vi "TDMS Merge Utility.vi"() -> ()   [LabVIEW 2011]
uses:
  <userlib>/_OpenG.lib/file/file.llb/Strip Path - Traditional__ogtk.vi
  <userlib>/_OpenG.lib/file/file.llb/Build Path - Traditional__ogtk.vi
  <userlib>/_OpenG.lib/file/file.llb/File Exists - Scalar__ogtk.vi
  <userlib>/_OpenG.lib/file/file.llb/Convert File Extension (Path)__ogtk.vi
panel:
  out "of":i32
  out "Files Processed":i32
  out "Progress Bar":u8(slide)=100 scale=0.0..100.0
  out "error out":errorcluster
  in  "Data Directory":path=path "\\\\10.196.0.53\\e$/Spartan/data/TDM"
  in  "Directory to Move":path=path "\\\\10.196.0.53\\e$/Spartan/data/xtdm"
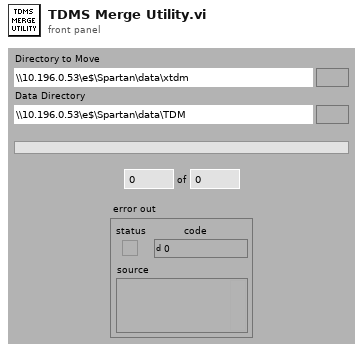
[diagram p1: front panel]
types:
  T1 = enum16{"open", "open or create", "create or replace", "create", "open (read-only)"}
  T2 = cluster{dbl, "tdms file out":refnum<k34>, string}
  T3 = cluster{dbl, "tdms file out":refnum<k34>, string}[]
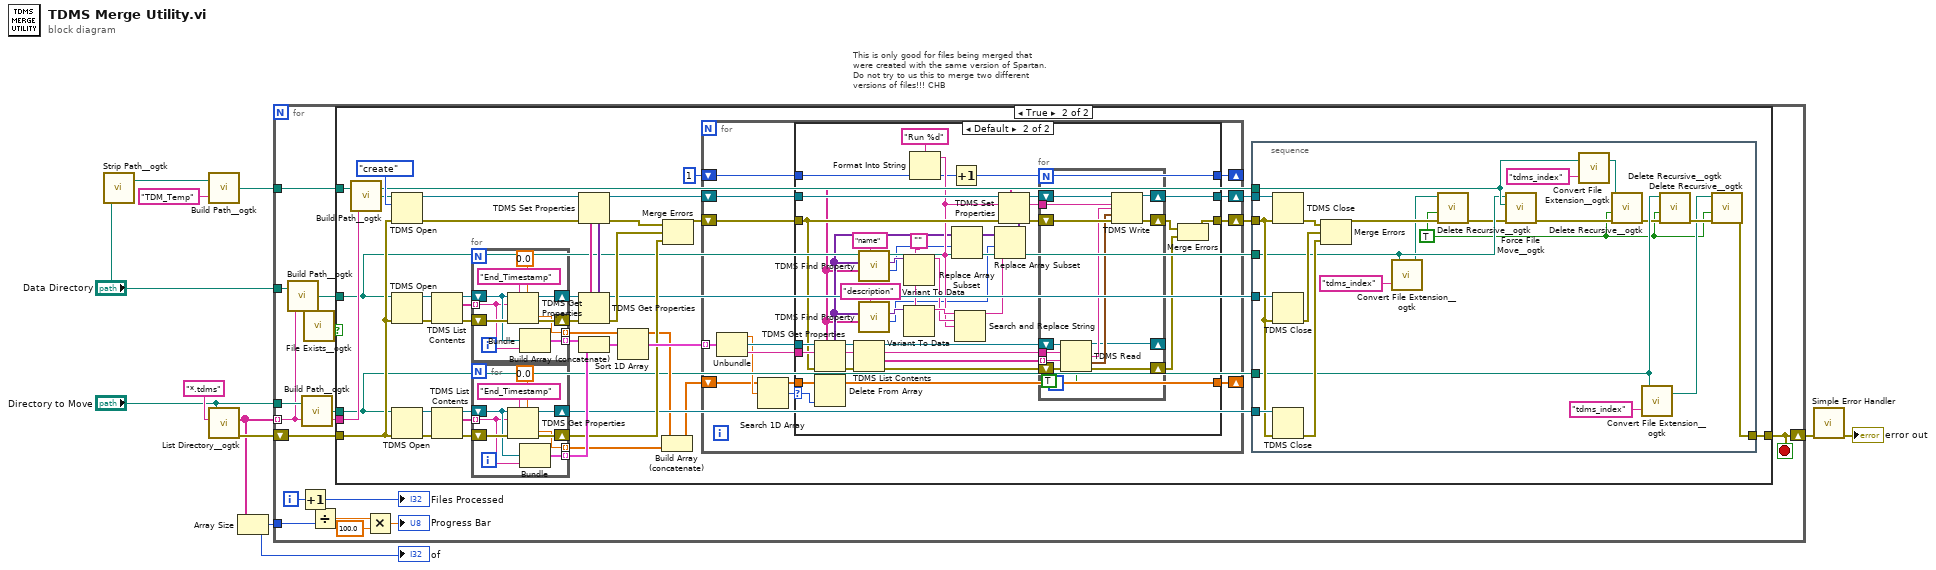
[diagram p0: block diagram]
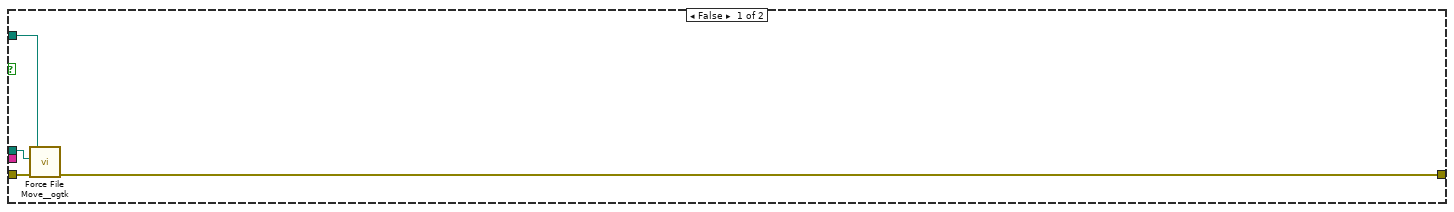
[diagram p2: hidden frame]
diagram:
  # "This is only good for files being merged that\nwere created with the same version of Spartan.\nDo not try to us this to merge two different\nversions of files!!! CHB"
  n1 = call-poly <userlib>:"Strip Path__ogtk.vi"("path"="Data Directory") -> ("stripped path"=w3:path)  [unwired: 1 out]
  n2 = call-poly <userlib>:"Build Path__ogtk.vi"("name or relative path"="TDM_Temp" ("Relative Path (\"\" - Folder)"), "base path"=w3) -> ("appended path"=w7:path)
  n3 = call <userlib>:"List Directory__ogtk.vi"("pattern"="*.tdms", "directory path"="Directory to Move") -> ("error out"=w10:errorcluster, "file names"=w2:string[])  [unwired: 2 in, 2 out]
  n4 = Array Size(array=w2) -> (size(s)=w1:i32)
  "of" <- w1
  n5 = for {
    shift-right: [w21] -> w6
    shift-left: w10 -> [w26]
    tunnel: w2 -> [w13] mode=indexing
    tunnel: "Data Directory" -> [w25]
    tunnel: "Directory to Move" -> [w14]
    tunnel: w7 -> [w22]
    tunnel: w1 -> [w18]
    i -> [w20]
    stop <- w21 stop-if-true
    n6 = call-poly <userlib>:"Build Path__ogtk.vi"("name or relative path"=w13, "base path"=w25) -> ("appended path"=w24:path)
    n7 = Increment(x=w20) -> (x+1=w19:i32)
    "Files Processed" <- w19
    n8 = call-poly <userlib>:"Build Path__ogtk.vi"("name or relative path"=w13, "base path"=w14) -> ("appended path"=w12:path)
    n9 = call-poly <userlib>:"File Exists__ogtk.vi"("file path"=w24) -> ("exists"=w23:bool)  [unwired: 6 in, 1 out]
    n10 = Divide(x=w19, y=w18) -> (x/y=w17:dbl)
    n11 = case shown="True" w23 {
      tunnel: w26 -> [w30 w66]
      tunnel: w13 -> [_ w64]
      tunnel: w24 -> [w29 w38]
      tunnel: [w28 w37] -> w21
      tunnel: w22 -> [_ w39]
      tunnel: w12 -> [w27 w31]
      frame False {
        n12 = call <userlib>:"Force File Move__ogtk.vi"("error in (no error)"=w30, "source"=w27, "target"=w29) -> ("error out"=w28:errorcluster)  [unwired: 3 in, 1 out]
      }
      frame True {
        n13 = call-poly <userlib>:"Build Path__ogtk.vi"("name or relative path"=w64, "base path"=w39) -> ("appended path"=w36:path)
        n14 = TDMS Open(8:w66, 10:T1."create" ("operation (0:open)"), 11:w36) -> (0:w53:errorcluster, 3:w52:refnum<k34>)  [unwired: 3 in]
        n15 = TDMS Open(8:w66, 11:w38) -> (0:w63:errorcluster, 3:w62:refnum<k34>)  [unwired: 4 in]
        n16 = TDMS Open(8:w66, 11:w31) -> (0:w71:errorcluster, 3:w70:refnum<k34>)  [unwired: 4 in]
        n17 = TDMS List Contents(4:w63, 7:w62) -> (0:w61:errorcluster, 2:w59:string[], 3:w60:refnum<k34>)  [unwired: 1 in, 1 out]
        n18 = TDMS List Contents(4:w71, 7:w70) -> (0:w69:errorcluster, 2:w67:string[], 3:w68:refnum<k34>)  [unwired: 1 in, 1 out]
        n19 = for {
          shift-right: [w171] -> w54
          shift-left: w61 -> [w173]
          shift-right: [w170] -> w55
          shift-left: w60 -> [w169]
          tunnel: w59 -> [w168] mode=indexing
          tunnel: [w167] -> w58 mode=indexing
          tunnel: [w165] -> w35 mode=indexing
          n20 = TDMS Get Properties(5:0.0, 7:"End_Timestamp" ("pattern"), 8:w173, 10:w168, 11:w169) -> (0:w171:errorcluster, 3:w170:refnum<k34>, 4:w165:dbl)  [unwired: 1 in, 3 out]
          n21 = Bundle(w165, "tdms file out"=w169, w168) -> (w167:T2)  [unwired: 1 in]
        }
        n22 = for {
          shift-right: [w180] -> w46
          shift-left: w69 -> [w182]
          shift-right: [w179] -> w40
          shift-left: w68 -> [w178]
          tunnel: w67 -> [w177] mode=indexing
          tunnel: [w176] -> w57 mode=indexing
          tunnel: [w174] -> w34 mode=indexing
          n23 = TDMS Get Properties(5:0.0, 7:"End_Timestamp" ("pattern"), 8:w182, 10:w177, 11:w178) -> (0:w180:errorcluster, 3:w179:refnum<k34>, 4:w174:dbl)  [unwired: 1 in, 3 out]
          n24 = Bundle(w174, "tdms file out"=w178, w177) -> (w176:T2)  [unwired: 1 in]
        }
        n25 = TDMS Get Properties(8:w54, 11:w55) -> (0:w47:errorcluster, 3:w41:refnum<k34>, 4:w50:variant[], 6:w51:string[])  [unwired: 4 in, 2 out]
        n26 = TDMS Set Properties(5:w50, 7:w51, 8:w53, 11:w52) -> (0:w45:errorcluster, 3:w48:refnum<k34>)  [unwired: 2 in, 2 out]
        n27 = Build Array (concatenate)(w58, w57) -> (w56:T3)
        n28 = Sort 1D Array(array=w56) -> (sorted array=w49:T3)
        n29 = Build Array (concatenate)(w35, w34) -> (w33:dbl[])
        n30 = Merge Errors(w45, w47, w46) -> (w44:errorcluster)
        n31 = for {
          tunnel: w49 -> [w107] mode=indexing
          shift-right: [w102] -> w42
          shift-left: w44 -> [w104]
          shift-right: [w101] -> w43
          shift-left: w48 -> [w103]
          shift-right: [w98] -> _
          shift-left: w33 -> [w97]
          shift-right: [w95] -> _
          shift-left: 1 -> [w96]
          n32 = Unbundle(w107) -> (w100:dbl, "tdms file out"=w106:refnum<k34>, w105:string)
          n33 = Search 1D Array(1D array=w97, element=w100) -> (index of element=w99:i32)  [unwired: 1 in]
          n34 = case shown="Default" w99 {
            selector: w99 -> [_ w114]
            tunnel: w106 -> [_ w149]
            tunnel: w105 -> [_ w148]
            tunnel: w104 -> [w111 w147]
            tunnel: w103 -> [w110 w146]
            tunnel: [w111 w134] -> w102
            tunnel: [w110 w132] -> w101
            tunnel: [w109 w115] -> w98
            tunnel: w97 -> [w109 w116]
            tunnel: w96 -> [w108 w113]
            tunnel: [w108 w112] -> w95
            frame -1 {
            }
            frame Default {
              w126 = ""
              n35 = TDMS Get Properties(8:w147, 10:w148, 11:w149) -> (0:w145:errorcluster, 2:w143:string, 3:w144:refnum<k34>, 4:w123:variant[], 6:w122:string[])  [unwired: 3 in, 1 out]
              n36 = Delete From Array(array=w116, index=w114) -> (array with subset deleted=w115:dbl[])  [unwired: 1 in, 1 out]
              n37 = TDMS List Contents(4:w145, 6:w143, 7:w144) -> (0:w141:errorcluster, 1:w139:string[], 2:w140:string, 3:w142:refnum<k34>)
              n38 = call "TDMS Find Property.vi"("Property Name"="name", "Property Names"=w122, "Property Values"=w123) -> ("Index"=w120:i32, "Property Value"=w127:variant)  [unwired: 4 out]
              n39 = call "TDMS Find Property.vi"("Property Name"="description", "Property Names"=w122, "Property Values"=w123) -> ("Index"=w119:i32, "Property Value"=w129:variant)  [unwired: 4 out]
              n40 = Variant To Data(type=w126, Variant=w127) -> (data=w125:string)  [unwired: 1 in, 1 out]
              n41 = Variant To Data(type=w126, Variant=w129) -> (data=w128:string)  [unwired: 1 in, 1 out]
              n42 = Format Into String(format string="Run %d", w113) -> (resulting string=w124:string)  [unwired: 2 in, 1 out]
              n43 = Increment(x=w113) -> (x+1=w112:i32)
              n44 = Replace Array Subset(array=w123, new element=w124, index=w120) -> (w121:variant[])
              n45 = Search and Replace String(input string=w128, search string=w125, replace string=w124) -> (result string=w118:string)  [unwired: 5 in, 3 out]
              n46 = Replace Array Subset(array=w121, new element=w118, index=w119) -> (w117:variant[])
              n47 = TDMS Set Properties(5:w117, 7:w122, 8:w147, 10:w124, 11:w146) -> (0:w138:errorcluster, 2:w136:string, 3:w137:refnum<k34>)  [unwired: 1 in, 1 out]
              n48 = for {
                shift-right: [w155] -> _
                shift-left: w142 -> [w164]
                shift-right: [w154] -> w133
                shift-left: w141 -> [w163]
                tunnel: w140 -> [w162]
                tunnel: w139 -> [w161] mode=indexing
                shift-right: [w153] -> w132
                shift-left: w137 -> [w159]
                shift-right: [w152] -> w135
                shift-left: w138 -> [w160]
                tunnel: w136 -> [w158]
                n49 = TDMS Read(0:w164, 5:w162, 7:w161, 11:w163, 13:TRUE ("return channels in file order? (F)")) -> (4:w155:refnum<k34>, 8:w157:string, 10:w156:waveform(dbl), 15:w154:errorcluster)  [unwired: 3 in, 2 out]
                n50 = TDMS Write(0:w159, 5:w158, 7:w157, 9:w156, 11:w160) -> (4:w153:refnum<k34>, 15:w152:errorcluster)  [unwired: 1 in, 2 out]
              }
              n51 = Merge Errors(w135, w133) -> (w134:errorcluster)
            }
          }
        }
        n52 = stacked-sequence {
          tunnel: w43 -> [w92]
          tunnel: w42 -> [w91]
          tunnel: w41 -> [w94]
          tunnel: w40 -> [w93]
          tunnel: w36 -> [w82]
          tunnel: w38 -> [w76]
          tunnel: w31 -> [w87]
          tunnel: [w78] -> w37
          frame #0 {
            w72 = TRUE ("Ignore Read-Only? (FALSE)")
            n53 = TDMS Close(8:w91, 11:w92) -> (0:w90:errorcluster)  [unwired: 1 out]
            n54 = TDMS Close(8:w91, 11:w94) -> (0:w89:errorcluster)  [unwired: 1 out]
            n55 = TDMS Close(8:w91, 11:w93) -> (0:w88:errorcluster)  [unwired: 1 out]
            n56 = Merge Errors(w90, w89, w88) -> (w75:errorcluster)
            n57 = call-poly <userlib>:"Convert File Extension__ogtk.vi"("new ending (none)"="tdms_index", "file name"=w76) -> ("new filename"=w73:path)  [unwired: 1 out]
            n58 = call <userlib>:"Delete Recursive__ogtk.vi"("error in (no error)"=w75, "Ignore Read-Only? (FALSE)"=w72, "Path"=w73) -> ("error out"=w74:errorcluster)  [unwired: 7 in, 1 out]
            n59 = call <userlib>:"Force File Move__ogtk.vi"("error in (no error)"=w74, "source"=w82, "target"=w76) -> ("error out"=w85:errorcluster)  [unwired: 3 in, 1 out]
            n60 = call-poly <userlib>:"Convert File Extension__ogtk.vi"("new ending (none)"="tdms_index", "file name"=w82) -> ("new filename"=w81:path)  [unwired: 1 out]
            n61 = call <userlib>:"Delete Recursive__ogtk.vi"("error in (no error)"=w85, "Ignore Read-Only? (FALSE)"=w72, "Path"=w81) -> ("error out"=w84:errorcluster)  [unwired: 7 in, 1 out]
            n62 = call-poly <userlib>:"Convert File Extension__ogtk.vi"("new ending (none)"="tdms_index", "file name"=w87) -> ("new filename"=w79:path)  [unwired: 1 out]
            n63 = call <userlib>:"Delete Recursive__ogtk.vi"("error in (no error)"=w84, "Ignore Read-Only? (FALSE)"=w72, "Path"=w87) -> ("error out"=w80:errorcluster)  [unwired: 7 in, 1 out]
            n64 = call <userlib>:"Delete Recursive__ogtk.vi"("error in (no error)"=w80, "Ignore Read-Only? (FALSE)"=w72, "Path"=w79) -> ("error out"=w78:errorcluster)  [unwired: 7 in, 1 out]
          }
        }
      }
    }
    n65 = Multiply(x=w17, y=100.0) -> (x*y=→"Progress Bar":dbl)
  }
  n66 = call <vilib>:"Simple Error Handler.vi"("error in (no error)"=w6) -> ("error out"=→"error out":errorcluster)  [unwired: 4 in, 4 out]
